vi "2D FFT and IFFT Functional Global.vi"(6 "FFT Dimension":enum16{"1D FFT", "2D FFT"}(ring)=enum."2D FFT", 7 "FFT States":T2(ring), 8 "Error In":errorcluster, 9 "Real In":dbl[][][](array[numeric]), 10 "Dimension FFT":cluster{"Depth":u64, "Height":u64, "Width":u64}={"Depth"=1, "Height"=1000, "Width"=1024} {"Width" min=1; "Height" min=1; "Depth" min=1}, 11 "Device":T1) -> (0 "Error Out":errorcluster, 2 "Labview Data":dbl[][](array[numeric]), 3 "OpenCLV Data":dbl[][](array[numeric]), 4 "Labview Time":u32, 5 "OpenCLV Time":u32)   [LabVIEW 2012]
uses:
  Non-User VIs/Controls/Device ID.ctl
  FFT Global.ctl
  Non-User VIs/FFT/FFT Control.ctl
  Non-User VIs/FFT/FFT Types.ctl
  Non-User VIs/FFT/FFT Dimension.ctl
  Non-User VIs/Controls/Memory Object.ctl
  Non-User VIs/Controls/Memory ID.ctl
  User Controls/Array Dimensions.ctl
  Non-User VIs/Controls/Memory Type.ctl
  Non-User VIs/FFT/FFT Direction.ctl
  Non-User VIs/Write Memory/WriteMemory_64f.vi
  Non-User VIs/FFT/Compute FFT 64f.vi
  Non-User VIs/Read Memory/ReadMemory_64f.vi
  <vilib>/Analysis/2dsp.llb/2D Real FFT.vi
  <vilib>/Analysis/2dsp.llb/2D Inverse Real FFT.vi
  <vilib>/Analysis/2dsp.llb/Real FFT.vi
  <vilib>/Analysis/2dsp.llb/Inverse Real FFT.vi
  Non-User VIs/FFT/Delete FFT Plan 64f.vi
  Non-User VIs/Allocate Memory/AllocateMemory_64f.vi
  Non-User VIs/FFT/Create FFT Plan 64f.vi
  OpenCLV x64.lvlib
  <vilib>/Analysis/NI_AALPro.lvlib
panel:
  in  "FFT Dimension 2":enum16{"1D FFT", "2D FFT"}(ring)=enum."2D FFT"
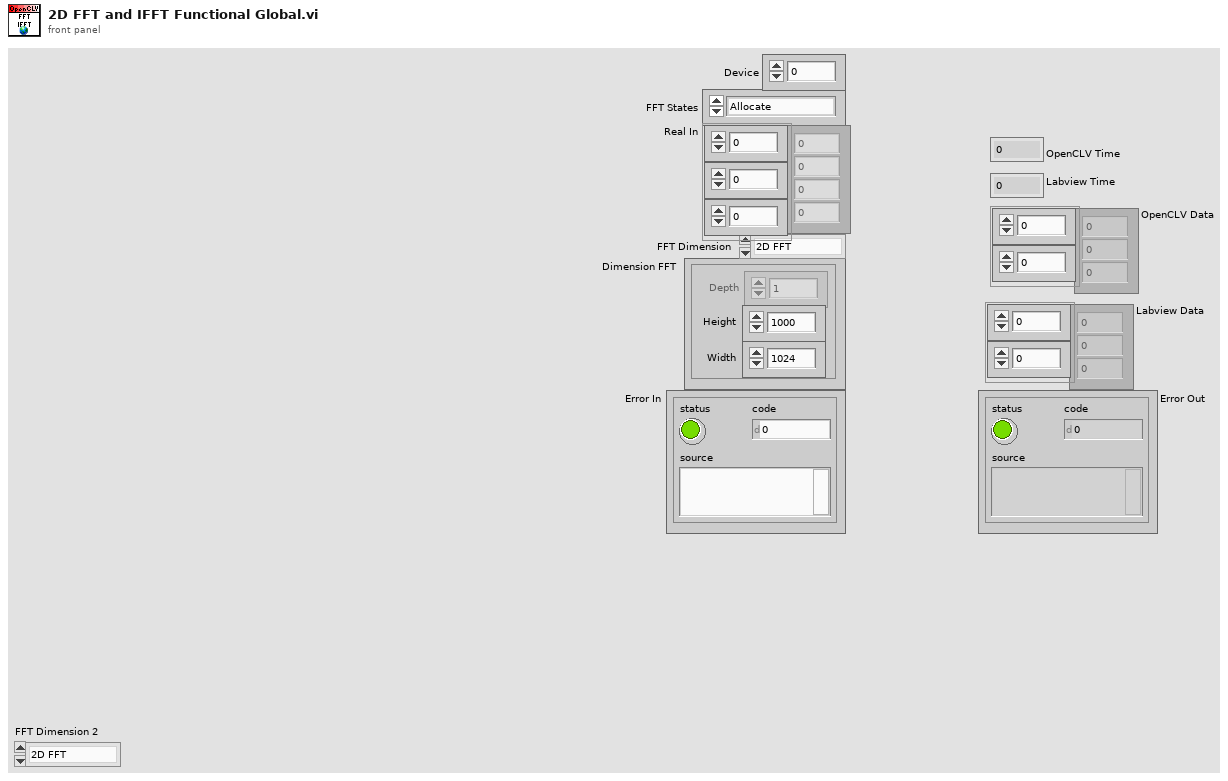
[diagram p1: front panel]
types:
  T1 = typedef "OpenCLV x64.lvlib/Device ID.ctl" = u64
  T2 = enum16{"Allocate", "Compute FFT and IFFT", "Compute Labivew FFT and IFFT", "Clean up"}
  T3 = typedef "FFT Global.ctl" = cluster{"FFT Object":T4, "IFFT Object":T4, "Memory Object":T7}
  T4 = typedef "OpenCLV x64.lvlib/FFT Control.ctl" = cluster{"Device ID":T1, "FFT Types":T5, "FFT Dim":T6, "Real":T7, "Imag":T7, "FFT Plan":u64, "FFT Direction":T11}
  T5 = typedef "OpenCLV x64.lvlib/FFT Types.ctl" = enum16{"Real to Hermitian", "Hermitian to Real", "Complex to Complex"}
  T6 = typedef "OpenCLV x64.lvlib/FFT Dimension.ctl" = enum16{"1D FFT", "2D FFT", "3D FFT"}
  T7 = typedef "OpenCLV x64.lvlib/Memory Object.ctl" = cluster{"Device ID":T1, "Memeroy ID":T8, "Dimension":T9, "Memory Type":T10}
  T8 = typedef "OpenCLV x64.lvlib/Memory ID.ctl" = u64
  T9 = typedef "Array Dimensions.ctl" = cluster{"Depth":u64, "Height":u64, "Width":u64}
  T10 = typedef "OpenCLV x64.lvlib/Memory Type.ctl" = enum16{"32f", "u8", "i8", "u16", "i16", "u32", "i32", "64f"}
  T11 = typedef "OpenCLV x64.lvlib/FFT Direction.ctl" = enum16{"Forward", "Reverse"}
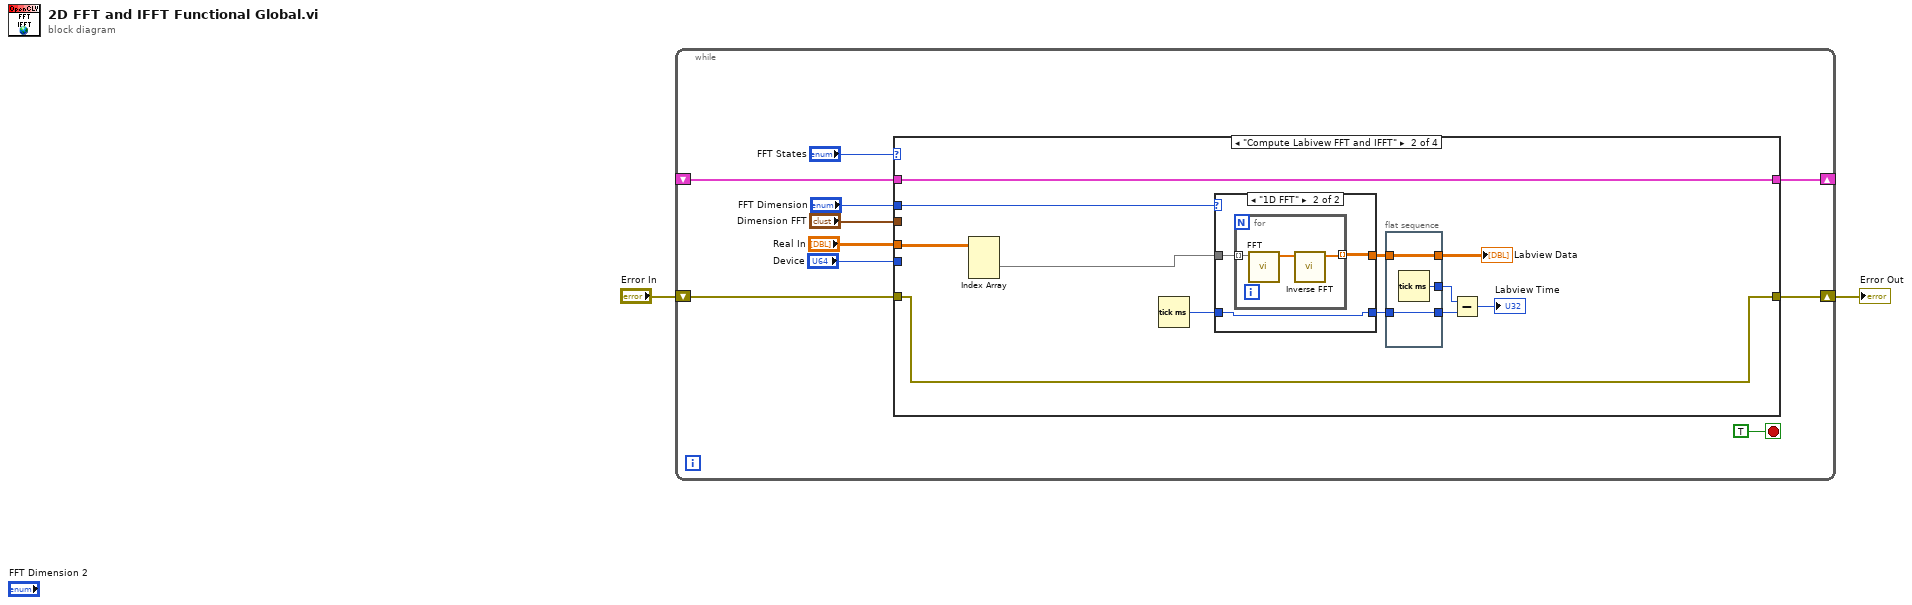
[diagram p0: block diagram]
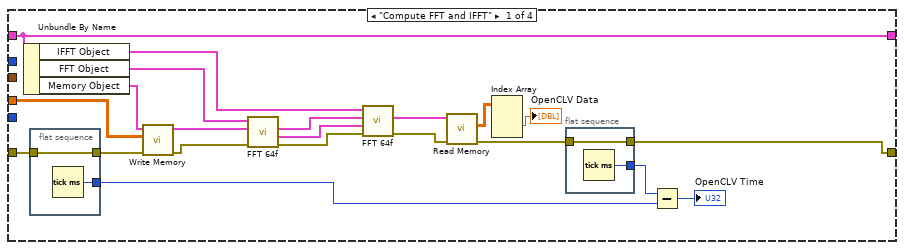
[diagram p2: hidden frame]
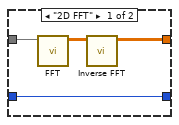
[diagram p3: hidden frame]
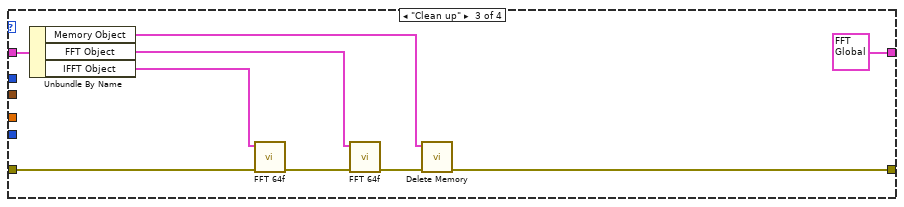
[diagram p4: hidden frame]
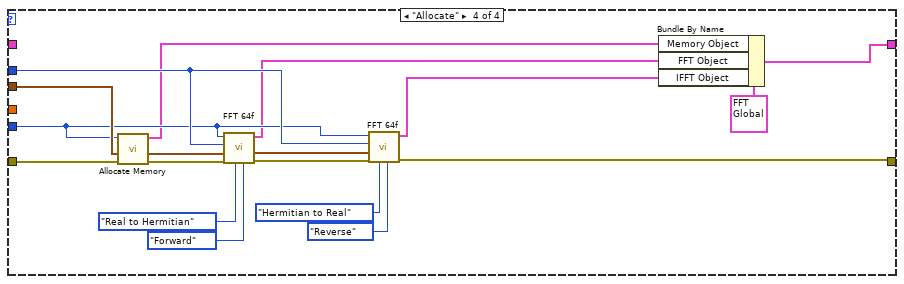
[diagram p5: hidden frame]
diagram:
  n1 = while {
    shift-right: [w6] -> w1
    shift-left: "Error In" -> [w7]
    shift-right: [w5] -> _
    shift-left: _ -> [w4]
    stop <- TRUE stop-if-true
    n2 = case shown="\"Compute Labivew FFT and IFFT\"" "FFT States" {
      tunnel: "Dimension FFT" -> [_ _ _ w89]
      tunnel: "FFT Dimension" -> [_ w49 _ w79]
      tunnel: "Device" -> [_ _ _ w78]
      tunnel: w7 -> [w19 w46 w71 w88]
      tunnel: [w15 w46 w64 w72] -> w6
      tunnel: [w31 w38 T3 {"FFT Object"={"Device ID"=0, "FFT Types"=enum."Real to Hermitian", "FFT Dim"=enum."1D FFT", "Real"={"Device ID"=0, "Memeroy ID"=0, "Dimension"={"Depth"=0, "Height"=0, "Width"=0}, "Memory Type"=enum."32f"}, "Imag"={"Device ID"=0, "Memeroy ID"=0, "Dimension"={"Depth"=0, "Height"=0, "Width"=0}, "Memory Type"=enum."32f"}, "FFT Plan"=0, "FFT Direction"=enum."Forward"}, "IFFT Object"={"Device ID"=0, "FFT Types"=enum."Real to Hermitian", "FFT Dim"=enum."1D FFT", "Real"={"Device ID"=0, "Memeroy ID"=0, "Dimension"={"Depth"=0, "Height"=0, "Width"=0}, "Memory Type"=enum."32f"}, "Imag"={"Device ID"=0, "Memeroy ID"=0, "Dimension"={"Depth"=0, "Height"=0, "Width"=0}, "Memory Type"=enum."32f"}, "FFT Plan"=0, "FFT Direction"=enum."Forward"}, "Memory Object"={"Device ID"=0, "Memeroy ID"=0, "Dimension"={"Depth"=1, "Height"=1, "Width"=1}, "Memory Type"=enum."32f"}} ("Global Variable Locals") w87] -> w5
      tunnel: w4 -> [w31 w38 w70 _]
      tunnel: "Real In" -> [w33 w48 _ _]
      frame "Compute FFT and IFFT" {
        n3 = Unbundle By Name(w31) -> ("IFFT Object"=w25:T4, "FFT Object"=w30:T4, "Memory Object"=w32:T7)
        n4 = flat-sequence {
          tunnel: [w35] -> w20
          tunnel: w19 -> [w35]
          tunnel: [w34] -> w14
          frame #0 {
            n5 = Tick Count (ms)() -> (millisecond timer value=w34:u32)
          }
        }
        n6 = call-poly "Write Memory.vi"("Error In"=w20, "Data In"=w33, "Memory Object In"=w32) -> ("Error Out"=w28:errorcluster, "Memory Object Out"=w29:T7)  [unwired: 6 in, 1 out]
        n7 = call-poly "FFT 64f.vi"("Error In"=w28, "Real In"=w29, "FFT Object"=w30) -> ("Error Out"=w18:errorcluster, "Imag Out"=w27:T7, "Real Out"=w26:T7)  [unwired: 4 in, 2 out]
        n8 = call-poly "FFT 64f.vi"("Error In"=w18, "Complex In"=w27, "Real In"=w26, "FFT Object"=w25) -> ("Error Out"=w17:errorcluster, "Real Out"=w23:T7)  [unwired: 3 in, 3 out]
        n9 = call-poly "Read Memory.vi"("Error In"=w17, "Memory Object In"=w23) -> ("Error Out"=w16:errorcluster, "Data Out"=w22:dbl[][][])  [unwired: 6 in, 2 out]
        n10 = Index Array(array=w22) -> (element=→"OpenCLV Data":dbl[][])  [unwired: 3 in]
        n11 = flat-sequence {
          tunnel: w16 -> [w37]
          tunnel: [w37] -> w15
          tunnel: [w36] -> w24
          frame #0 {
            n12 = Tick Count (ms)() -> (millisecond timer value=w36:u32)
          }
        }
        n13 = Subtract(x=w24, y=w14) -> (x-y=→"OpenCLV Time":u32)
      }
      frame "Compute Labivew FFT and IFFT" {
        n14 = Index Array(array=w48) -> (element=w47:dbl[][])  [unwired: 3 in]
        n15 = Tick Count (ms)() -> (millisecond timer value=w45:u32)
        n16 = case shown="\"1D FFT\"" w49 {
          tunnel: w47 -> [w56 w59]
          tunnel: [w55 w58] -> w43
          tunnel: w45 -> [w53 w57]
          tunnel: [w53 w57] -> w42
          frame "2D FFT" {
            n17 = call-poly <vilib>:"FFT.vi"("X"=w56) -> ("FFT {X}"=w54:cdb[][])  [unwired: 9 in, 1 out]
            n18 = call-poly <vilib>:"Inverse FFT.vi"("FFT {X}"=w54) -> ("X"=w55:dbl[][])  [unwired: 9 in, 1 out]
          }
          frame "1D FFT" {
            n19 = for {
              tunnel: w59 -> [w62] mode=indexing
              tunnel: [w61] -> w58 mode=indexing
              n20 = call-poly <vilib>:"FFT.vi"("X"=w62) -> ("FFT {X}"=w60:cdb[])  [unwired: 9 in, 1 out]
              n21 = call-poly <vilib>:"Inverse FFT.vi"("FFT {X}"=w60) -> ("X"=w61:dbl[])  [unwired: 9 in, 1 out]
            }
          }
        }
        n22 = flat-sequence {
          tunnel: [w52] -> w44
          tunnel: w43 -> [w52]
          tunnel: w42 -> [w51]
          tunnel: [w51] -> w41
          tunnel: [w50] -> w40
          frame #0 {
            n23 = Tick Count (ms)() -> (millisecond timer value=w50:u32)
          }
        }
        n24 = Subtract(x=w40, y=w41) -> (x-y=→"Labview Time":u32)
        "Labview Data" <- w44
      }
      frame "Clean up" {
        n25 = Unbundle By Name(w70) -> ("Memory Object"=w65:T7, "FFT Object"=w67:T4, "IFFT Object"=w69:T4)
        n26 = call-poly "FFT 64f.vi"("Error In"=w71, "FFT Object"=w69) -> ("Error Out"=w68:errorcluster)  [unwired: 9 in]
        n27 = call-poly "FFT 64f.vi"("Error In"=w68, "FFT Object"=w67) -> ("Error Out"=w66:errorcluster)  [unwired: 9 in]
        n28 = call "Delete Memory.vi"("Error In"=w66, "Memory Object In"=w65) -> ("Error Out"=w64:errorcluster)  [unwired: 8 in, 1 out]
      }
      frame "Allocate" {
        n29 = call-poly "Allocate Memory.vi"("Error In"=w88, "Dimension"=w89, "Device In"=w78) -> ("Error Out"=w85:errorcluster, "Dimensions Out"=w84:T9, "Memory Object"=w75:T7)  [unwired: 6 in]
        n30 = call-poly "FFT 64f.vi"("Direction"=FFT_Direction."Forward", "FFT Types"=FFT_Types."Real to Hermitian", "Error In"=w85, "Dimension"=w84, "FFT Dimension"=w79, "Labview Device"=w78) -> ("Error Out"=w83:errorcluster, "FFT Output Dimensions"=w80:T9, "FFT Object"=w74:T4)  [unwired: 3 in]
        n31 = call-poly "FFT 64f.vi"("Direction"=FFT_Direction."Reverse", "FFT Types"=FFT_Types."Hermitian to Real", "Error In"=w83, "Dimension"=w80, "FFT Dimension"=w79, "Labview Device"=w78) -> ("Error Out"=w72:errorcluster, "FFT Object"=w73:T4)  [unwired: 3 in, 1 out]
        n32 = Bundle By Name(cluster=T3 {"FFT Object"={"Device ID"=0, "FFT Types"=enum."Real to Hermitian", "FFT Dim"=enum."1D FFT", "Real"={"Device ID"=0, "Memeroy ID"=0, "Dimension"={"Depth"=0, "Height"=0, "Width"=0}, "Memory Type"=enum."32f"}, "Imag"={"Device ID"=0, "Memeroy ID"=0, "Dimension"={"Depth"=0, "Height"=0, "Width"=0}, "Memory Type"=enum."32f"}, "FFT Plan"=0, "FFT Direction"=enum."Forward"}, "IFFT Object"={"Device ID"=0, "FFT Types"=enum."Real to Hermitian", "FFT Dim"=enum."1D FFT", "Real"={"Device ID"=0, "Memeroy ID"=0, "Dimension"={"Depth"=0, "Height"=0, "Width"=0}, "Memory Type"=enum."32f"}, "Imag"={"Device ID"=0, "Memeroy ID"=0, "Dimension"={"Depth"=0, "Height"=0, "Width"=0}, "Memory Type"=enum."32f"}, "FFT Plan"=0, "FFT Direction"=enum."Forward"}, "Memory Object"={"Device ID"=0, "Memeroy ID"=0, "Dimension"={"Depth"=1, "Height"=1, "Width"=1}, "Memory Type"=enum."32f"}} ("Global Variable Locals"), "Memory Object"=w75, "FFT Object"=w74, "IFFT Object"=w73) -> (w87:T3)
      }
    }
  }
  "Error Out" <- w1
